vi "test6.2-RegisterInterruptFromNonCSM.vi"(8 "error in (no error)":errorcluster, 11 "TestCase in":refnum<class "testcase-CSMBroadcast.lvclass">) -> (0 "error out":errorcluster, 3 "TestCase out":refnum<class "testcase-CSMBroadcast.lvclass">)   [LabVIEW 2017, in "testcase-CSMBroadcast.lvclass"]
uses:
  testcase-CSMBroadcast.lvclass
  <vilib>/addons/_JKI Toolkits/VI Tester/TestCase.llb/TestCase.lvclass
  src/user.lib/_NEVSTOP/Communicable State Machine(CSM)/Communicable State Machine.lvlib
  CSM/CSM-Testcase.lvlib
  C:/Program Files (x86)/National Instruments/LabVIEW 2017/vi.lib/addons/_JKI Toolkits/VI Tester/TestCase.llb/TestCase.lvclass
panel:
  out "output cluster":T1
  out "LoopCount":i32
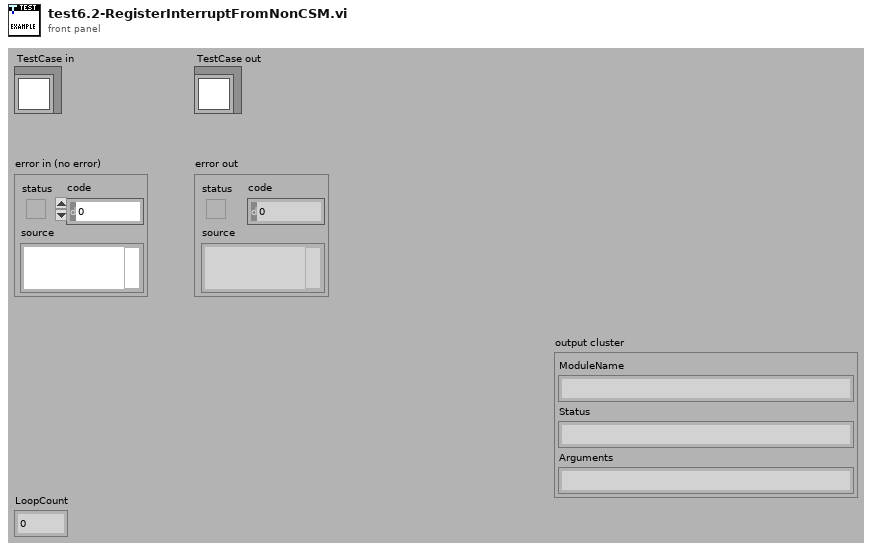
[diagram p1: front panel]
types:
  T1 = cluster{"ModuleName":string, "Status":string, "Arguments":string}
  T2 = cluster{"Status Event":refnum<user-event>, "Interrupt Event":refnum<user-event>}
  T3 = cluster{"cluster":cluster{"ModuleName":string, "Status":string, "Arguments":string}}
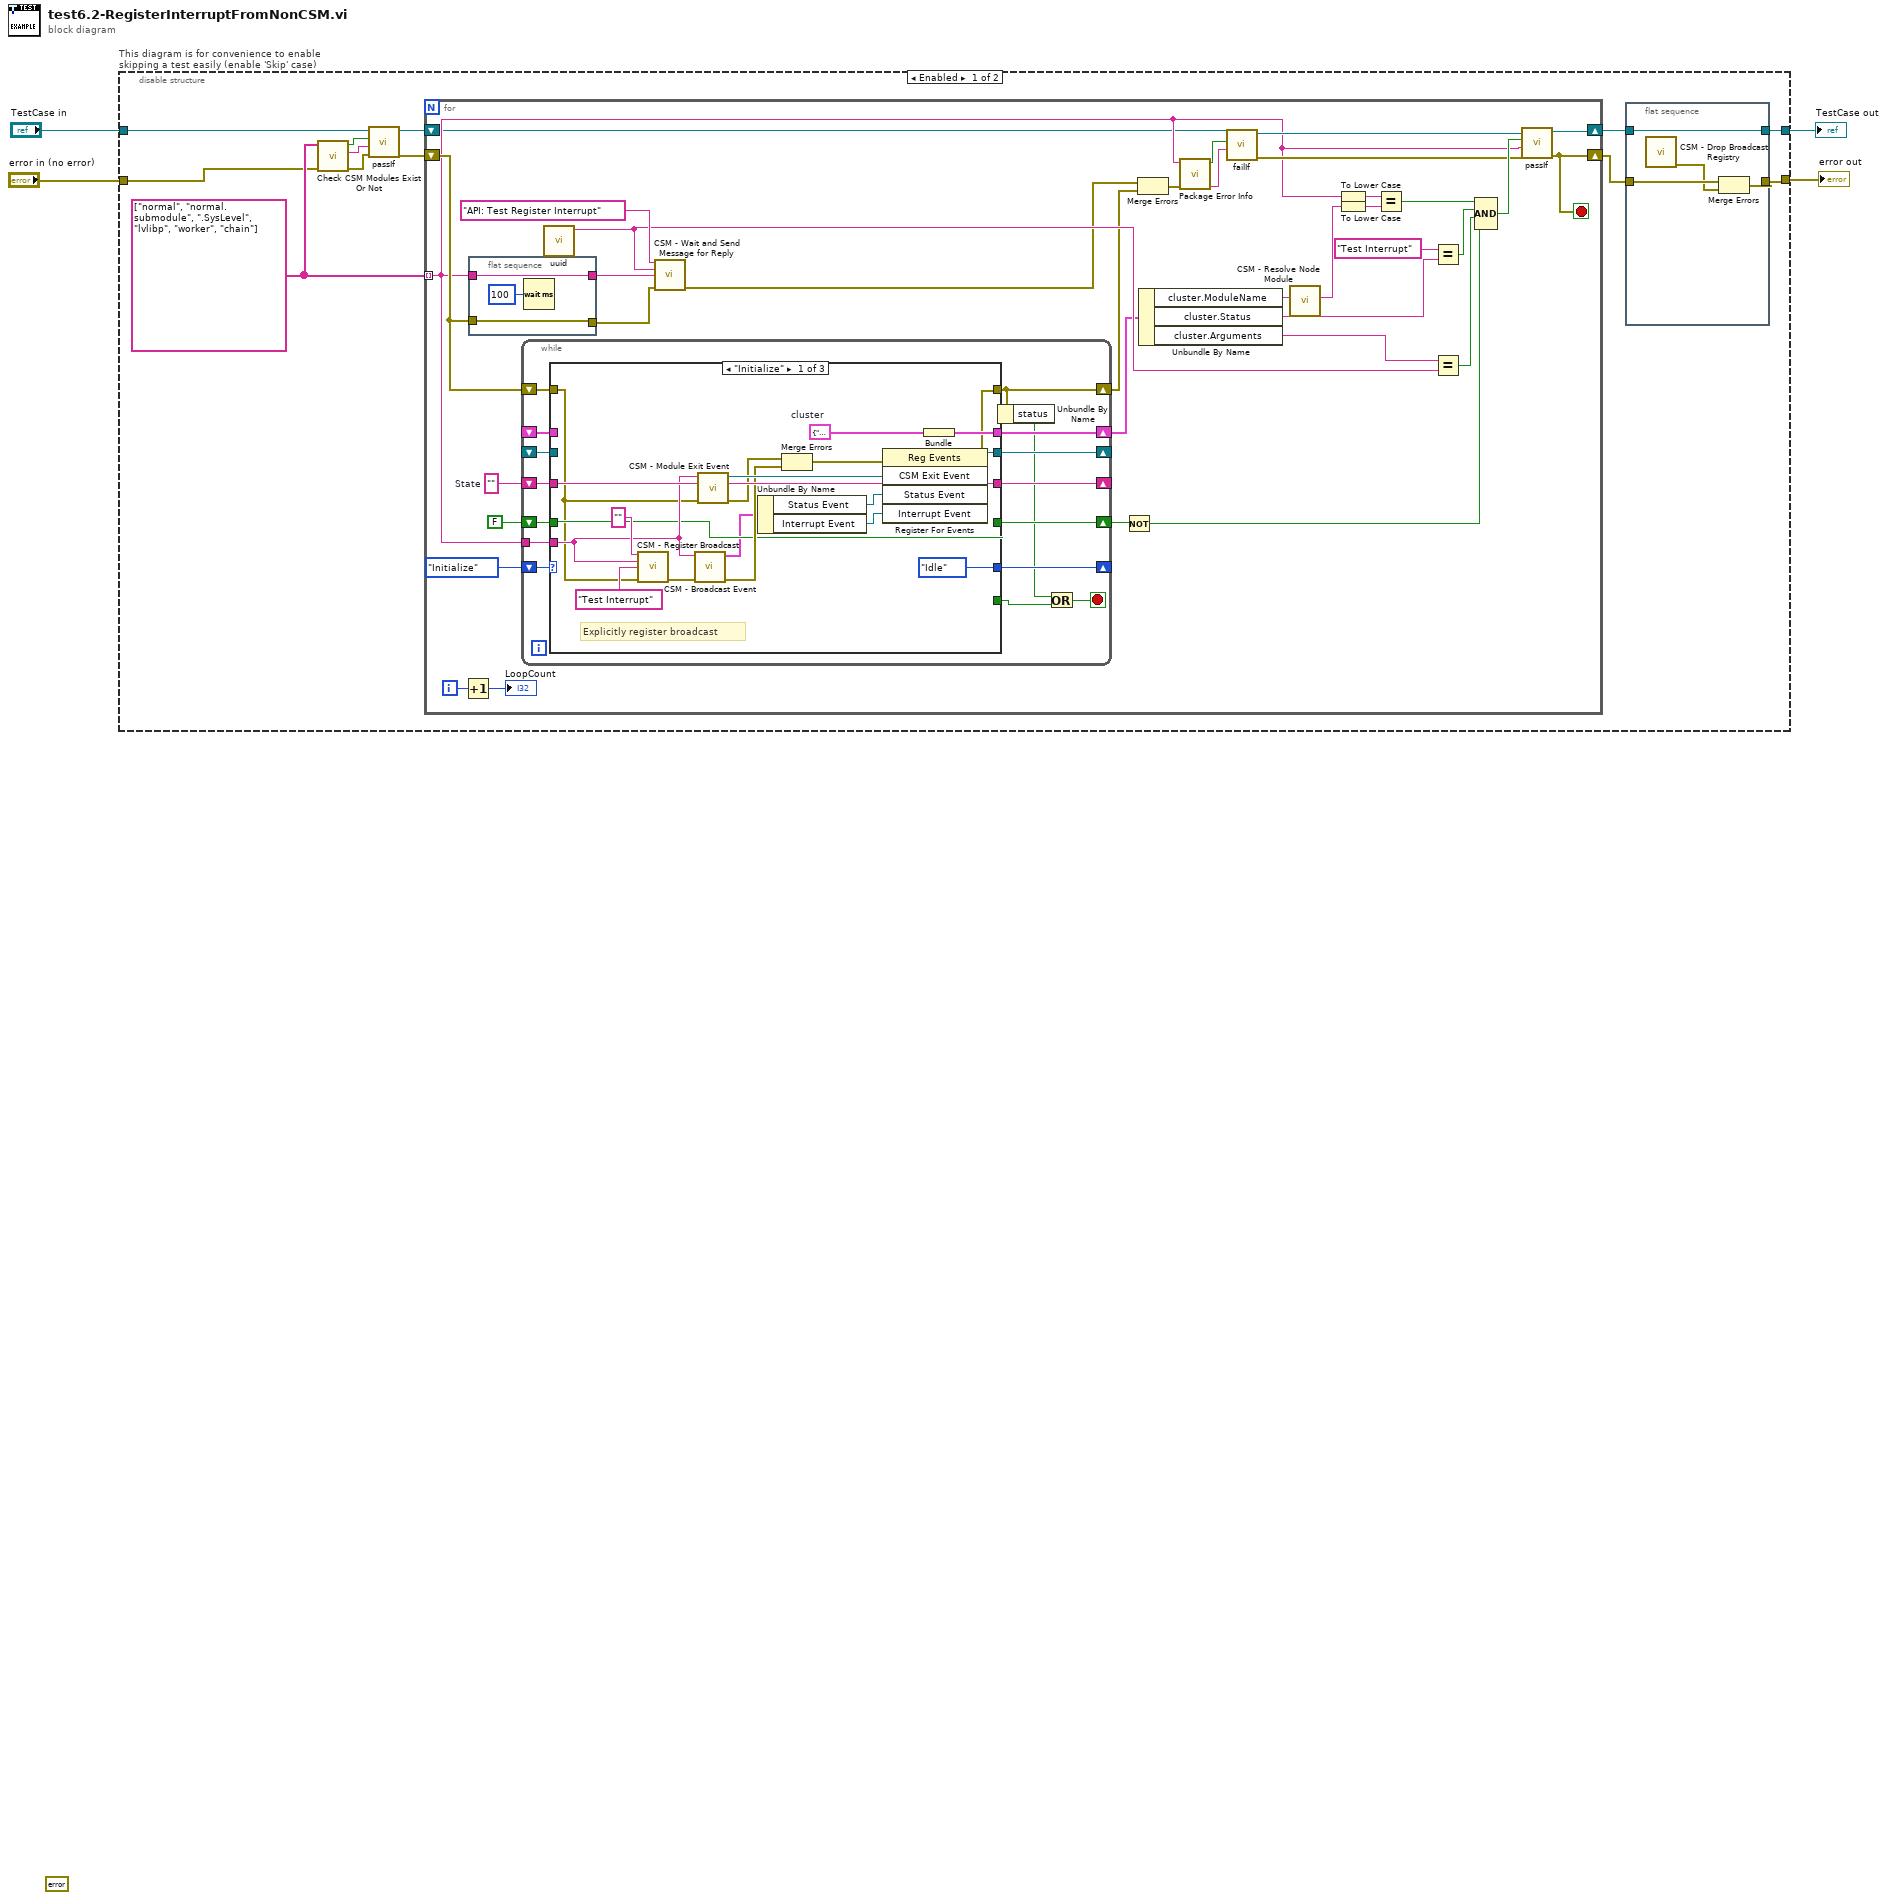
[diagram p0: block diagram]
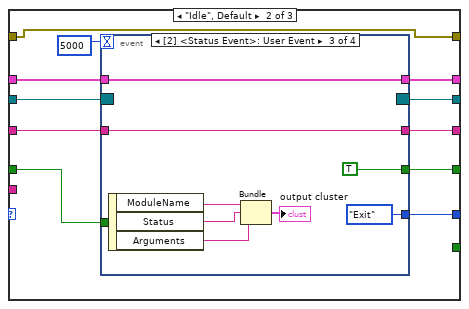
[diagram p2: hidden frame]
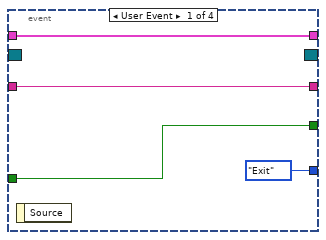
[diagram p3: hidden frame]
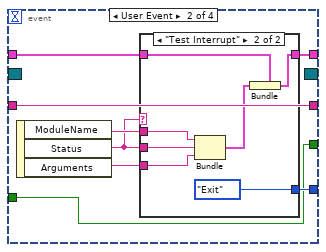
[diagram p4: hidden frame]
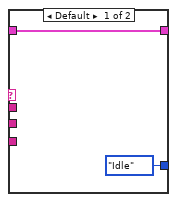
[diagram p5: hidden frame]
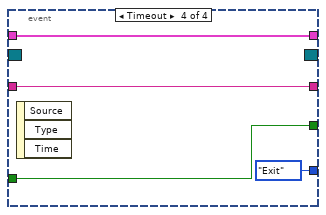
[diagram p6: hidden frame]
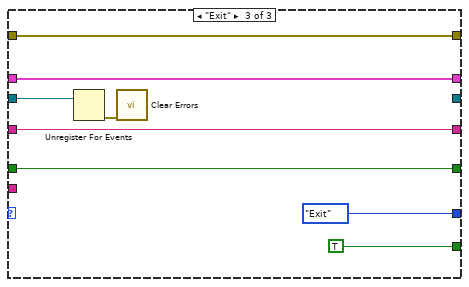
[diagram p7: hidden frame]
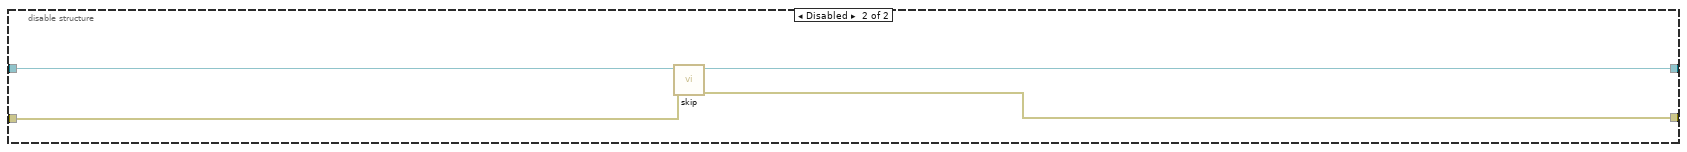
[diagram p8: hidden frame]
diagram:
  (unwired) errorcluster {"status"=FALSE, "code"=0, "source"=""} ("error out")
  n1 = disable-structure "This diagram is for convenience to enable skipping a test easily (enable 'Skip' case)" shown="Enabled" {
    disable-tunnel: "TestCase in" -> [w11 w149]
    disable-tunnel: [w6 w147] -> w2
    disable-tunnel: [w16 w148] -> w1
    disable-tunnel: "error in (no error)" -> [w8 w146]
    frame Enabled {
      w12 = string[] ["normal", "normal.submodule", ".SysLevel", "lvlibp", "worker", "chain"]
      n2 = call "Check CSM Modules Exist Or Not.vi"("error in"=w8, "CSM names in"=w12) -> ("error out"=w13:errorcluster, "Debug string"=w14:string, "All Modules Exist?"=w15:bool)  [unwired: 7 in]
      n3 = call-dynamic "passIf.vi"("error in (no error)"=w13, "message (\"\")"=w14, "pass"=w15, "TestCase in"=w11) -> ("error out"=w9:errorcluster, "TestCase out"=w10:refnum<class "testcase-CSMBroadcast.lvclass">)  [unwired: 6 in]
      n4 = for {
        shift-right: [w47] -> w7
        shift-left: w10 -> [w21]
        tunnel: w12 -> [w22] mode=indexing
        shift-right: [w40] -> w5
        shift-left: w9 -> [w30]
        i -> [w42]
        stop <- w40 stop-if-true
        w54 = ""  # State
        n5 = Increment(x=w42) -> (x+1=→"LoopCount":i32)
        n6 = flat-sequence {
          tunnel: w22 -> [w58]
          tunnel: [w58] -> w52
          tunnel: w30 -> [w56]
          tunnel: [w56] -> w31
          frame #0 {
            n7 = Wait (ms)(milliseconds to wait=u32 100) -> ()  [unwired: 1 out]
          }
        }
        n8 = while {
          shift-right: [w73] -> _
          shift-left: enum16{"Idle", "Initialize", "Exit"}."Initialize" -> [w74]
          shift-right: [w71] -> _
          shift-left: w54 -> [w72]
          shift-right: [w70] -> _
          shift-left: _ -> [w69]
          shift-right: [w68] -> w39
          shift-left: _ -> [w67]
          tunnel: w22 -> [w66]
          shift-right: [w65] -> w34
          shift-left: FALSE -> [w64]
          shift-right: [w60] -> w24
          shift-left: w30 -> [w63]
          stop <- w62 stop-if-true
          n9 = case shown="\"Initialize\"" w74 {
            tunnel: [enum16{"Idle", "Initialize", "Exit"}."Idle" w104 enum16{"Idle", "Initialize", "Exit"}."Exit"] -> w73
            tunnel: [_ _ TRUE] -> w61
            tunnel: w72 -> [w92 w102 w143]
            tunnel: [w92 w103 w143] -> w71
            tunnel: [w90 w100 _] -> w70
            tunnel: w69 -> [_ w101 w142]
            tunnel: [w89 w98 w140] -> w68
            tunnel: w67 -> [_ w99 w140]
            tunnel: w66 -> [w82 _ _]
            tunnel: [w79 w96 w139] -> w65
            tunnel: w64 -> [w79 w95 w139]
            tunnel: w63 -> [w77 w94 w138]
            tunnel: [w75 w94 w138] -> w60
            frame "Initialize" {
              w88 = T1 {"ModuleName"="", "Status"="", "Arguments"=""}  # cluster
              # "Explicitly register broadcast"
              n10 = call "CSM - Register Broadcast.vi"("CSM Name(Empty for Broadcast Event)"="", "Source CSM Name (* as Default)"=w82, "Trigger"="Test Interrupt" ("State"), "Error In"=w77) -> ("error out"=w84:errorcluster)  [unwired: 10 in, 1 out]
              n11 = call "CSM - Broadcast Event.vi"("Error In"=w84, "CSM Module"=w82) -> ("error out"=w86:errorcluster, "Broadcast Event"=w78:T2)  [unwired: 7 in, 1 out]
              n12 = call "CSM - Module Exit Event.vi"("Error In"=w77, "Name (\"\" to Use UUID) In"=w82) -> ("error out"=w87:errorcluster, "CSM Exit Event"=w91:refnum<user-event>)  [unwired: 7 in, 1 out]
              n13 = Unbundle By Name(w78) -> ("Status Event"=w81:refnum<user-event>, "Interrupt Event"=w80:refnum<user-event>)
              n14 = Merge Errors(w87, w86) -> (w76:errorcluster)
              n15 = register-events(error in=w76, w91, w81, w80) -> (reference out=w90:refnum<event-registration>, error out=w75:errorcluster)  [unwired: 1 in]
              n16 = Bundle("cluster"=w88) -> (w89:T3)  [unwired: 1 in]
            }
            frame "Idle", Default {
              n17 = event shown="[2] <Status Event>: User Event" {
                selector: w101 -> [_ _ _ _]
                dyn-events: [_ _ _ _] -> w100
                timeout: 5000 -> [_ _ _ _]
                tunnel: [enum16{"Idle", "Initialize", "Exit"}."Exit" w115 enum16{"Idle", "Initialize", "Exit"}."Exit" enum16{"Idle", "Initialize", "Exit"}."Exit"] -> w104
                tunnel: w102 -> [w108 w116 w133 w137]
                tunnel: [w108 w116 w133 w137] -> w103
                tunnel: w99 -> [w106 w112 w132 w136]
                tunnel: [w106 w111 w132 w136] -> w98
                tunnel: [w105 w109 TRUE w134] -> w96
                tunnel: w95 -> [w105 w109 _ w134]
                event User Event {
                  n18 = event-data() -> ()  [unwired: 1 in, 1 out]
                }
                event User Event {
                  n19 = event-data() -> ("ModuleName"=w114:string, "Status"=w110:string, "Arguments"=w113:string)  [unwired: 1 in]
                  n20 = case shown="\"Test Interrupt\"" w110 {
                    tunnel: [enum16{"Idle", "Initialize", "Exit"}."Idle" enum16{"Idle", "Initialize", "Exit"}."Exit"] -> w115
                    tunnel: w114 -> [_ w124]
                    tunnel: w110 -> [_ w123]
                    tunnel: w113 -> [_ w122]
                    tunnel: w112 -> [w118 w121]
                    tunnel: [w118 w119] -> w111
                    frame Default {
                    }
                    frame "Test Interrupt" {
                      n21 = Bundle("ModuleName"=w124, "Status"=w123, "Arguments"=w122) -> (w120:T1)  [unwired: 1 in]
                      n22 = Bundle(cluster=w121, "cluster"=w120) -> (w119:T3)
                    }
                  }
                }
                event User Event {
                  n23 = event-data() -> ("ModuleName"=w129:string, "Status"=w128:string, "Arguments"=w127:string)  [unwired: 1 in]
                  n24 = Bundle("ModuleName"=w129, "Status"=w128, "Arguments"=w127) -> (→"output cluster":T1)  [unwired: 1 in]
                }
                event Timeout {
                  n25 = event-data() -> ()  [unwired: 1 in, 3 out]
                }
              }
            }
            frame "Exit" {
              n26 = Unregister For Events(event registration refnum=w142) -> (error out=w141:errorcluster)  [unwired: 1 in]
              n27 = call <vilib>:"Clear Errors.vi"("error in (no error)"=w141) -> ()  [unwired: 5 in, 2 out]
            }
          }
          n28 = Unbundle By Name(w60) -> ("status"=w59:bool)
          n29 = Or(x=w59, y=w61) -> (x .or. y?=w62:bool)
        }
        n30 = call "uuid.vi"() -> ("UUID"=w49:string)  [unwired: 11 in]
        n31 = call "CSM - Wait and Send Message for Reply.vi"("State"="API: Test Register Interrupt", "Arguments (\"\")"=w49, "Target Module"=w52, "Error In (No Error)"=w31) -> ("error out"=w25:errorcluster)  [unwired: 8 in, 3 out]
        n32 = Not(x=w34) -> (.not. x?=w33:bool)
        n33 = Merge Errors(w25, w24) -> (w23:errorcluster)
        n34 = Unbundle By Name(w39) -> ("cluster.ModuleName"=w37:string, "cluster.Status"=w50:string, "cluster.Arguments"=w48:string)
        n35 = call "Package Error Info.vi"("error in"=w23, "String in"=w22) -> ("packed error info out"=w28:string, "error status"=w29:bool)  [unwired: 8 in]
        n36 = call-dynamic "failIf.vi"("message (\"\")"=w28, "fail"=w29, "TestCase in"=w21) -> ("error out"=w26:errorcluster, "TestCase out"=w27:refnum<class "testcase-CSMBroadcast.lvclass">)  [unwired: 7 in]
        n37 = call "CSM - Resolve Node Module.vi"("Node Name"=w37) -> ("CSM Module Name"=w35:string)  [unwired: 10 in]
        n38 = To Lower Case(string=w22) -> (all lower case string=w38:string)
        n39 = To Lower Case(string=w35) -> (all lower case string=w36:string)
        n40 = Equal?(x=w38, y=w36) -> (x = y?=w46:bool)
        n41 = Equal?(x="Test Interrupt" ("State"), y=w50) -> (x = y?=w45:bool)
        n42 = Equal?(x=w48, y=w49) -> (x = y?=w44:bool)
        n43 = Compound Arithmetic op=AND(w46, w45, w44, w33) -> (w43:bool)
        n44 = call-dynamic "passIf.vi"("error in (no error)"=w26, "message (\"\")"=w22, "pass"=w43, "TestCase in"=w27) -> ("error out"=w40:errorcluster, "TestCase out"=w47:refnum<class "testcase-CSMBroadcast.lvclass">)  [unwired: 6 in]
      }
      n45 = flat-sequence {
        tunnel: w5 -> [w20]
        tunnel: [w19] -> w16
        tunnel: w7 -> [w17]
        tunnel: [w17] -> w6
        frame #0 {
          n46 = call "CSM - Drop Broadcast Registry.vi"() -> ("error out"=w18:errorcluster)  [unwired: 15 in]
          n47 = Merge Errors(w20, w18) -> (w19:errorcluster)
        }
      }
    }
    frame Disabled {
      # "skip test result while test is under development"
      n48 = call <vilib>:"skip.vi"("error in (no error)"=w146, "TestCase in"=w149) -> ("error out"=w148:errorcluster, "TestCase out"=w147:refnum<class "testcase-CSMBroadcast.lvclass">)  [unwired: 8 in]
    }
  }
  "error out" <- w1
  "TestCase out" <- w2
